vi "SmartSEM Remote API save FIB probe table.vi"(8 "error in":errorcluster, 10 "FIB Probe":string(combo), 11 "Api":refnum<k7>(container)) -> (0 "error out":errorcluster, 3 "Api out":refnum<k7>)   [LabVIEW 2018]
uses:
  <vilib>/Utility/file.llb/Write To Spreadsheet File (string).vi
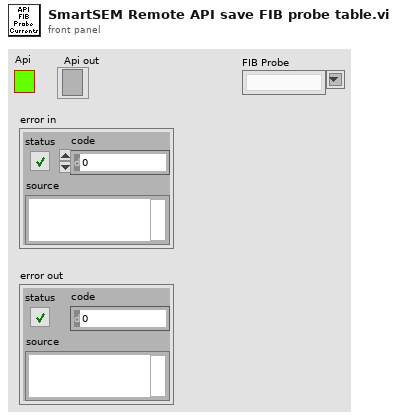
[diagram p1: front panel]
types:
  T1 = cluster{"FIB mode":u8, "FIB focus":sgl, "FIB probe current":sgl, "FIB emission current":sgl, "FIB rotation":sgl, "FIB aperture X":sgl, "FIB aperture Y":sgl, "FIB stig X":sgl, "FIB stig Y":sgl, "FIB beam shift X":sgl, "FIB beam shift Y":sgl}
  T2 = cluster{"Filament (A)":sgl, "Accelerator Target (V)":sgl, "Accelerator Actual (V)":sgl, "Extrator Target (V)":sgl, "Extrator Actual (V)":sgl, "Emission Target (uA)":sgl, "Emission Actual (uA)":sgl, "Suppressor (V)":sgl, "Faraday I (nA)":sgl, "Lens1 Target (V)":sgl, "Lens1 Actual (V)":sgl, "Lens2 Target (V)":sgl, "Lens2 Actual (V)":sgl, "Gun Vac (Torr)":sgl, "Column Vac (Torr)":sgl, "Tip Lifetime (uAhr)":sgl}
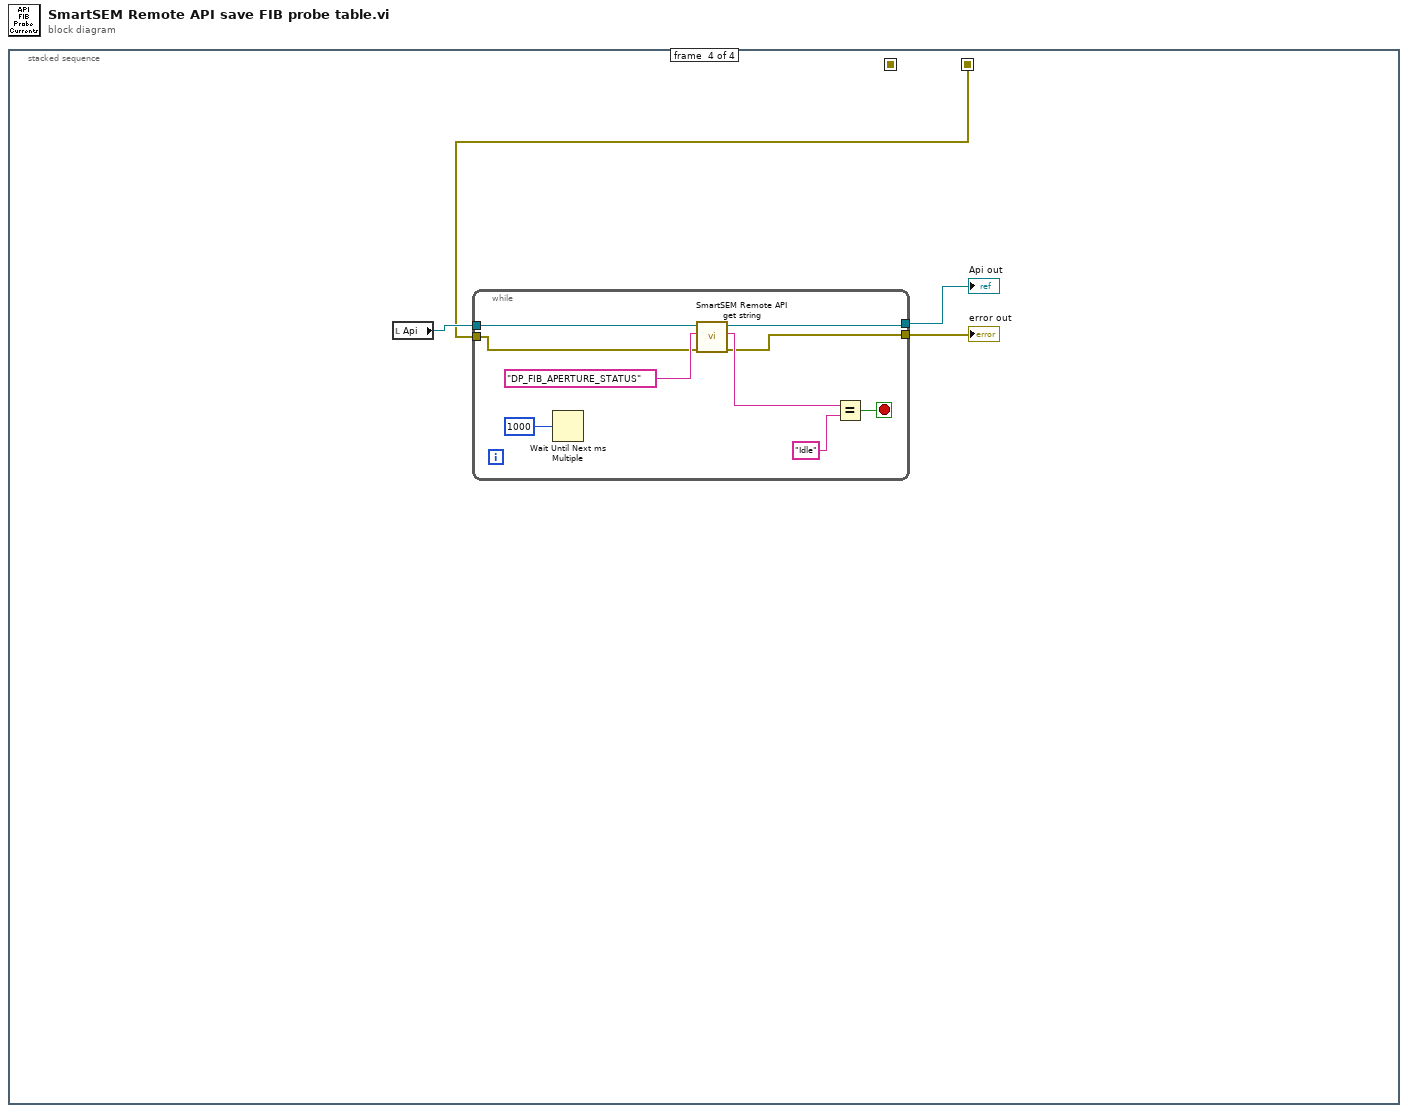
[diagram p0: block diagram]
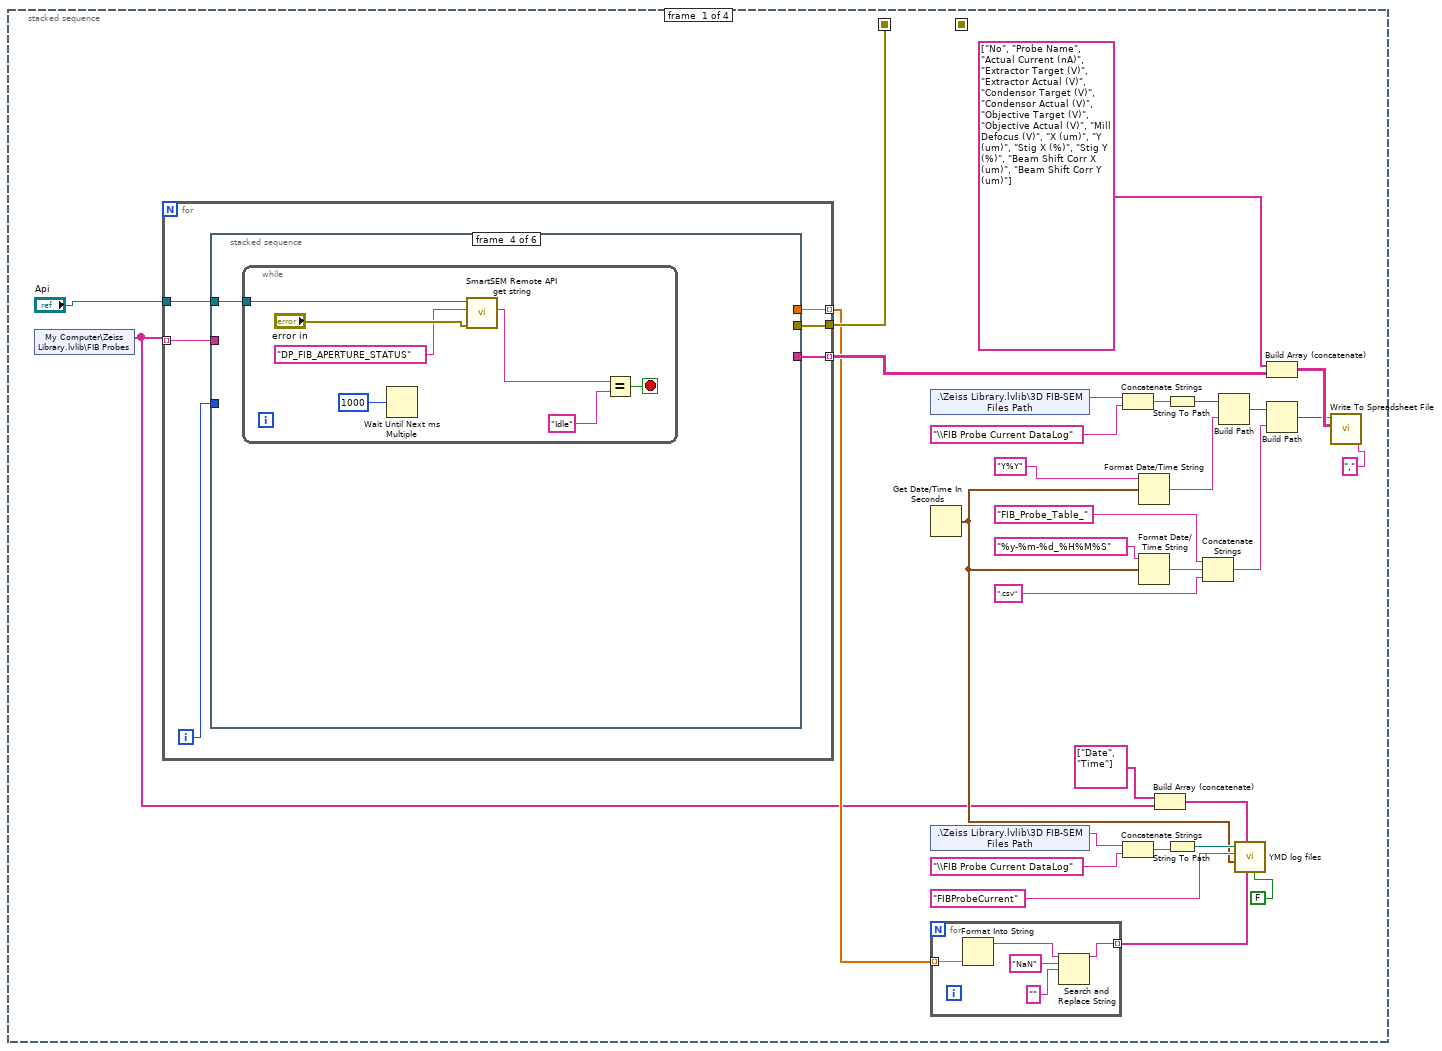
[diagram p2: hidden frame]
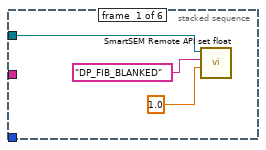
[diagram p3: hidden frame]
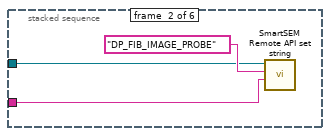
[diagram p4: hidden frame]
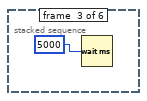
[diagram p5: hidden frame]
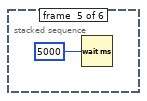
[diagram p6: hidden frame]
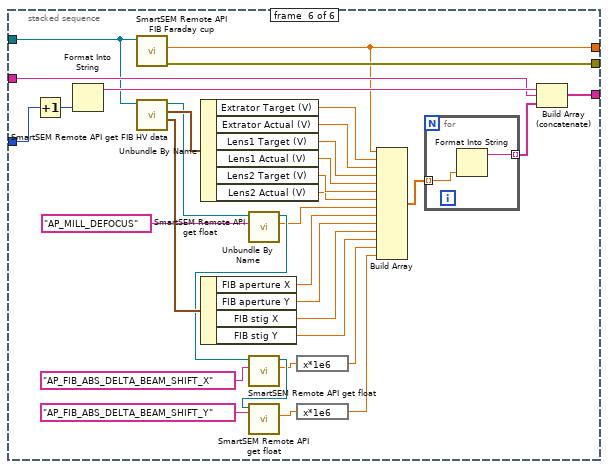
[diagram p7: hidden frame]
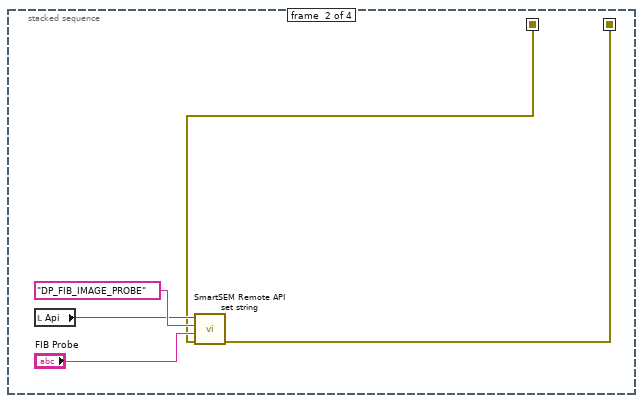
[diagram p8: hidden frame]
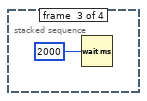
[diagram p9: hidden frame]
diagram:
  n1 = stacked-sequence {
    seq-local: [w19 _ _ _] -> [_ w95 _ _]
    seq-local: [_ w94 _ _] -> [_ _ _ w102]
    frame #0 {
      n2 = shared-variable "My Computer\\Zeiss Library.lvlib\\FIB Probes"() -> (w1:string[])  [unwired: 1 in, 1 out]
      n3 = for {
        tunnel: "Api" -> [w42]
        tunnel: [w41] -> w19
        tunnel: w1 -> [w40] mode=indexing
        tunnel: [w38] -> w31 mode=indexing
        tunnel: [w37] -> w3 mode=indexing
        i -> [w39]
        n4 = stacked-sequence {
          tunnel: w40 -> [_ w47 _ _ _ w87]
          tunnel: w42 -> [w43 w46 _ w50 _ w85]
          tunnel: [_ _ _ _ _ w91] -> w41
          tunnel: w39 -> [_ _ _ _ _ w90]
          tunnel: [_ _ _ _ _ w86] -> w38
          tunnel: [_ _ _ _ _ w70] -> w37
          frame #0 {
            n5 = call "SmartSEM Remote API set float.vi"("vValue"=sgl 1.0, "lpszParam"="DP_FIB_BLANKED", "Api"=w43) -> ()  [unwired: 7 in, 2 out]
          }
          frame #1 {
            n6 = call "SmartSEM Remote API set string.vi"("vValue"=w47, "lpszParam"="DP_FIB_IMAGE_PROBE", "Api"=w46) -> ()  [unwired: 7 in, 2 out]
          }
          frame #2 {
            n7 = Wait (ms)(milliseconds to wait=u32 5000) -> ()  [unwired: 1 out]
          }
          frame #3 {
            n8 = while {
              tunnel: w50 -> [w53]
              stop <- w55 stop-if-true
              n9 = Wait Until Next ms Multiple(millisecond multiple=u32 1000) -> ()  [unwired: 1 out]
              n10 = call "SmartSEM Remote API get string.vi"("error in"="error in", "lpszParam"="DP_FIB_APERTURE_STATUS", "Api"=w53) -> ("data"=w51:string)  [unwired: 6 in, 2 out]
              n11 = Equal?(x=w51, y="Idle" ("lpszParam")) -> (x = y?=w55:bool)
            }
          }
          frame #4 {
            n12 = Wait (ms)(milliseconds to wait=u32 5000) -> ()  [unwired: 1 out]
          }
          frame #5 {
            n13 = Increment(x=w90) -> (x+1=w89:i32)
            n14 = Format Into String(w89) -> (resulting string=w88:string)  [unwired: 3 in, 1 out]
            n15 = call "SmartSEM Remote API FIB Faraday cup.vi"("Api"=w85) -> ("error out"=w91:errorcluster, "FIB Faraday Cup (nA)"=w70:sgl)  [unwired: 8 in, 1 out]
            n16 = call "SmartSEM Remote API get FIB HV data.vi"("Api in"=w85) -> ("FIB parameters"=w83:T1, "Capella HV Data Output"=w84:T2, "Api out"=w62:refnum<k7>)  [unwired: 7 in, 1 out]
            n17 = Unbundle By Name(w84) -> ("Extrator Target (V)"=w73:sgl, "Extrator Actual (V)"=w82:sgl, "Lens1 Target (V)"=w81:sgl, "Lens1 Actual (V)"=w72:sgl, "Lens2 Target (V)"=w80:sgl, "Lens2 Actual (V)"=w71:sgl)
            n18 = Unbundle By Name(w83) -> ("FIB aperture X"=w79:sgl, "FIB aperture Y"=w78:sgl, "FIB stig X"=w77:sgl, "FIB stig Y"=w76:sgl)
            n19 = call "SmartSEM Remote API get float.vi"("lpszParam"="AP_MILL_DEFOCUS", "Api"=w62) -> ("vValue"=w60:sgl, "Api out"=w61:refnum<k7>)  [unwired: 7 in, 1 out]
            n20 = call "SmartSEM Remote API get float.vi"("lpszParam"="AP_FIB_ABS_DELTA_BEAM_SHIFT_X", "Api"=w61) -> ("vValue"=w66:sgl, "Api out"=w67:refnum<k7>)  [unwired: 7 in, 1 out]
            n21 = call "SmartSEM Remote API get float.vi"("lpszParam"="AP_FIB_ABS_DELTA_BEAM_SHIFT_Y", "Api"=w67) -> ("vValue"=w64:sgl)  [unwired: 7 in, 2 out]
            n22 = expression code="x*1e6"(w66) -> (w65:sgl)
            n23 = expression code="x*1e6"(w64) -> (w63:sgl)
            n24 = Build Array(w70, w73, w82, w81, w72, w80, w71, w60, w79, w78, w77, w76, w65, w63) -> (w75:sgl[])
            n25 = for {
              tunnel: w75 -> [w93] mode=indexing
              tunnel: [w92] -> w74 mode=indexing
              n26 = Format Into String(w93) -> (resulting string=w92:string)  [unwired: 3 in, 1 out]
            }
            n27 = Build Array (concatenate)(w88, w87, w74) -> (w86:string[])
          }
        }
      }
      n28 = shared-variable ".\\Zeiss Library.lvlib\\3D FIB-SEM Files Path"() -> (w23:string)  [unwired: 1 in, 1 out]
      n29 = Get Date/Time In Seconds() -> (seconds since 1Jan1904=w2:timestamp)
      n30 = shared-variable ".\\Zeiss Library.lvlib\\3D FIB-SEM Files Path"() -> (w7:string)  [unwired: 1 in, 1 out]
      n31 = for {
        tunnel: [w32] -> w8 mode=indexing
        tunnel: w3 -> [w36] mode=indexing
        n32 = Format Into String(w36) -> (resulting string=w33:string)  [unwired: 3 in, 1 out]
        n33 = Search and Replace String(input string=w33, search string="NaN", replace string="" ("replace string (\"\")")) -> (result string=w32:string)  [unwired: 5 in, 3 out]
      }
      n34 = Concatenate Strings(w23, "\\FIB Probe Current DataLog" ("Log file name")) -> (w22:string)
      n35 = Concatenate Strings(w7, "\\FIB Probe Current DataLog" ("Log file name")) -> (w5:string)
      n36 = Format Date/Time String(time format string (%c)="Y%Y", seconds (now)=w2) -> (date/time string=w27:string)  [unwired: 1 out]
      n37 = Format Date/Time String(time format string (%c)="%y-%m-%d_%H%M%S", seconds (now)=w2) -> (date/time string=w16:string)  [unwired: 1 out]
      n38 = Build Array (concatenate)(string[] ["Date", "Time"], w1) -> (w9:string[])
      n39 = String To Path(string=w22) -> (path=w25:path)
      n40 = String To Path(string=w5) -> (path=w4:path)
      n41 = Concatenate Strings("FIB_Probe_Table_" ("time format string (%c)"), w16, ".csv" ("time format string (%c)")) -> (w14:string)
      n42 = Build Path(base path=w25, name or relative path=w27) -> (appended path=w21:path)
      n43 = call "YMD log files.vi"("Day"=FALSE ("Month"), "Input text array"=w8, "Input header array"=w9, "current time"=w2, "Log file name"="FIBProbeCurrent", "Log file path"=w4) -> ()  [unwired: 6 in]
      n44 = Build Array (concatenate)(string[] ["No", "Probe Name", "Actual Current (nA)", "Extractor Target (V)", "Extractor Actual (V)", "Condensor Target (V)", "Condensor Actual (V)", "Objective Target (V)", "Objective Actual (V)", "Mill Defocus (V)", "X (um)", "Y (um)", "Stig X (%)", "Stig Y (%)", "Beam Shift Corr X (um)", "Beam Shift Corr Y (um)"], w31) -> (w29:string[][])
      n45 = Build Path(base path=w21, name or relative path=w14) -> (appended path=w20:path)
      n46 = call-poly <vilib>:"Write To Spreadsheet File.vi"("delimiter (\\t)"="," ("delimiter (\\t)"), "2D data"=w29, "file path (dialog if empty)"=w20) -> ()  [unwired: 5 in, 1 out]
    }
    frame #1 {
      n47 = local read "Api"() -> (w96:refnum<k7>)
      n48 = call "SmartSEM Remote API set string.vi"("error in"=w95, "vValue"="FIB Probe", "lpszParam"="DP_FIB_IMAGE_PROBE", "Api"=w96) -> ("error out"=w94:errorcluster)  [unwired: 6 in, 1 out]
    }
    frame #2 {
      n49 = Wait (ms)(milliseconds to wait=u32 2000) -> ()  [unwired: 1 out]
    }
    frame #3 {
      n50 = local read "Api"() -> (w103:refnum<k7>)
      n51 = while {
        tunnel: w103 -> [w109]
        tunnel: w102 -> [w106]
        tunnel: [w104] -> w101
        tunnel: [w105] -> w100
        stop <- w110 stop-if-true
        n52 = Wait Until Next ms Multiple(millisecond multiple=u32 1000) -> ()  [unwired: 1 out]
        n53 = call "SmartSEM Remote API get string.vi"("error in"=w106, "lpszParam"="DP_FIB_APERTURE_STATUS", "Api"=w109) -> ("error out"=w104:errorcluster, "data"=w107:string, "Api out"=w105:refnum<k7>)  [unwired: 6 in]
        n54 = Equal?(x=w107, y="Idle" ("lpszParam")) -> (x = y?=w110:bool)
      }
      "Api out" <- w100
      "error out" <- w101
    }
  }
